vi "Set Trigger ID.vi"(10 "Trigger ID":u8, 11 "TimerDRV in":refnum<class "TimerDRV.lvclass">) -> (3 "TimerDRV out":refnum<class "TimerDRV.lvclass">)   [LabVIEW 2019, in "TimingDRV Engine.lvlib" / "TimerDRV.lvclass"]
uses:
  TimerDRV.lvclass
  TimerDRV.lvclass/TimerDRV.ctl
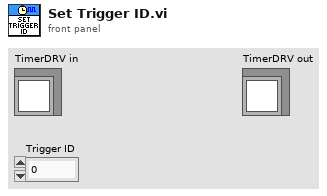
[diagram p1: front panel]
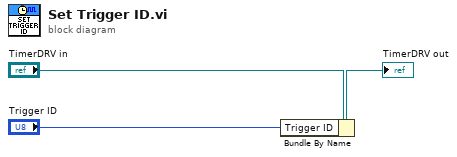
[diagram p0: block diagram]
diagram:
  n1 = Bundle By Name(cluster="TimerDRV in", "Trigger ID"="Trigger ID") -> (→"TimerDRV out":refnum<class "TimerDRV.lvclass">)
